vi "PhotonPipelineResult_Unpack.vi"(11 "RawData":u8[](array[numeric])) -> (3 "PhotonPipelineResult_REF":T1)   [LabVIEW 2019, in "PhotonVisionLib.lvlib"]
doc: "Internal function to parse the data returned by PhotonCamera_GetLatestResult.\n\nInputs:\n - RawData -- Byte array containing the data to parse.\n\nOutputs:\n - PipelineResult -- Parsed PipelineResult cluster."
uses:
  PhotonVisionLib.lvlib
  TargetCorner_New.vi
  Packet_decode_Int32.vi
  Packet_decode_Transform3d.vi
  PhotonPNPResult_unpackt.vi
  PhotonMultiTargetPNPResult_New.vi
  PhotonMultiTargetPNPResult_MAX_IDS.vi
  Packet_decode_Int16.vi
  <vilib>/Rock Robotics/WPI/ThirdParty/JAS_Junk/TrajLib/VI/Transform3d_Create_Trans3dRot3d.vi
  <vilib>/Rock Robotics/WPI/ThirdParty/JAS_Junk/TrajLib/VI/Translation3d_Create.vi
  <vilib>/Rock Robotics/WPI/ThirdParty/JAS_Junk/TrajLib/VI/Rotation3d_Create_Quaternion.vi
  <vilib>/Rock Robotics/WPI/ThirdParty/JAS_Junk/TrajLib/VI/Quaternion_New.vi
  Packet_decode_Boolean.vi
  PhotonPNPResult_New_Empty.vi
  PhotonPNPResult_New.vi
  <vilib>/Rock Robotics/WPI/ThirdParty/JAS_Junk/TrajLib/VI/Quaternion_Normalize.vi
  <vilib>/Rock Robotics/WPI/ThirdParty/JAS_Junk/TrajLib/VI/Quaternion_New_Default.vi
  TypeDef/TargetCornerType.ctl
  TypeDef/PhotonTrackedTargetType.ctl
  <vilib>/Rock Robotics/WPI/ThirdParty/JAS_Junk/TrajLib/TypeDef/QUATERNION.ctl
  <vilib>/Rock Robotics/WPI/ThirdParty/JAS_Junk/TrajLib/Trajectory_Library.lvlib
  <vilib>/Rock Robotics/WPI/ThirdParty/JAS_Junk/TrajLib/TypeDef/ROTATION3D.ctl
  <vilib>/Rock Robotics/WPI/ThirdParty/JAS_Junk/TrajLib/TypeDef/TRANSLATION3D.ctl
  <vilib>/Rock Robotics/WPI/ThirdParty/JAS_Junk/TrajLib/TypeDef/TRANSFORM3D.ctl
  TypeDef/PhotonPNPResultType.ctl
  TypeDef/PhotonMultiTargetPNPResultType.ctl
  TypeDef/PhotonPipelineResultType.ctl
  Ref/PhotonPipelineResult_REF.ctl
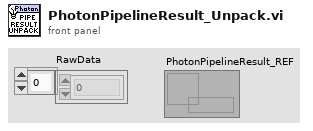
[diagram p1: front panel]
types:
  T1 = typedef "PhotonVisionLib.lvlib/PhotonPipelineResult_REF.ctl" = refnum<data-value>
  T2 = typedef "PhotonVisionLib.lvlib/PhotonMultiTargetPNPResultType.ctl" = cluster{"PhotonPNPResult":T3, "FiducialIDsUsed":i16[]}
  T3 = typedef "PhotonVisionLib.lvlib/PhotonPNPResultType.ctl" = cluster{"IsPresent":bool, "bestReprojErr":dbl, "altReprojErr":dbl, "ambiguity":dbl, "Best":T4, "Alt":T4}
  T4 = typedef "Trajectory_Library.lvlib/TRANSFORM3D.ctl" = cluster{"TRANSLATION3D":T5, "ROTATION3D":T6, "XF":bool}
  T5 = typedef "Trajectory_Library.lvlib/TRANSLATION3D.ctl" = cluster{"X":dbl, "Y":dbl, "Z":dbl}
  T6 = typedef "Trajectory_Library.lvlib/ROTATION3D.ctl" = cluster{"Q_quaternion":T7}
  T7 = typedef "Trajectory_Library.lvlib/QUATERNION.ctl" = cluster{"R":dbl, "V":dbl[]}
  T8 = typedef "PhotonVisionLib.lvlib/PhotonTrackedTargetType.ctl" = cluster{"Yaw":dbl, "Pitch":dbl, "Area":dbl, "Skew":dbl, "MinAreaRectCorners":T9[], "BestCameraToTarget":T4, "FiiducialId":i32, "AltCameraToTarget":T4, "PoseAmbiguity":dbl, "DetectedCorners":T9[]}
  T9 = typedef "PhotonVisionLib.lvlib/TargetCornerType.ctl" = cluster{"X":dbl, "Y":dbl}
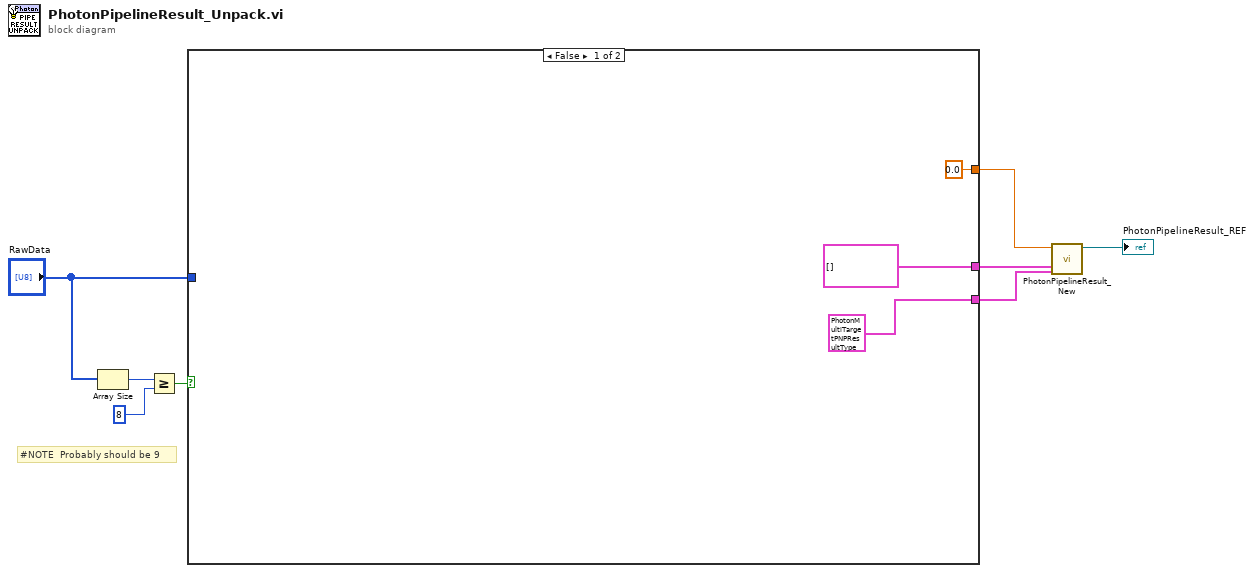
[diagram p0: block diagram]
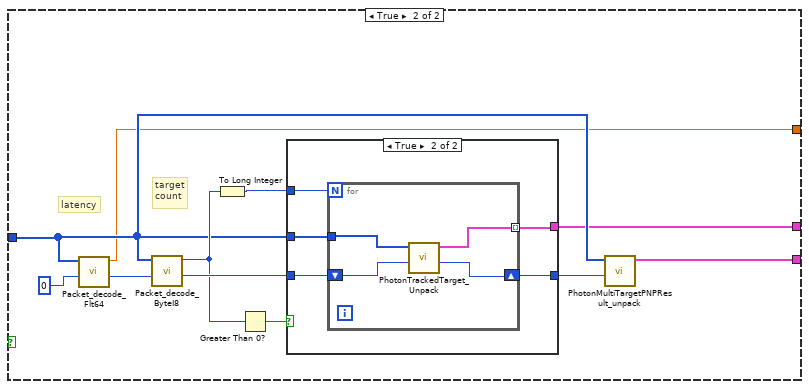
[diagram p2: hidden frame]
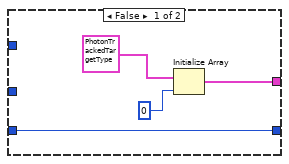
[diagram p3: hidden frame]
diagram:
  # "#NOTE  Probably should be 9"
  n1 = Array Size(array="RawData") -> (size(s)=w7:i32)
  n2 = Greater Or Equal?(x=w7, y=8) -> (x >= y?=w8:bool)
  n3 = case shown="False" w8 {
    tunnel: "RawData" -> [_ w15]
    tunnel: [T2 {"PhotonPNPResult"={"IsPresent"=FALSE, "bestReprojErr"=0.0, "altReprojErr"=0.0, "ambiguity"=0.0, "Best"={"TRANSLATION3D"={"X"=0.0, "Y"=0.0, "Z"=0.0}, "ROTATION3D"={"Q_quaternion"={"R"=1.0, "V"=[0.0, 0.0, 0.0]}}, "XF"=FALSE}, "Alt"={"TRANSLATION3D"={"X"=0.0, "Y"=0.0, "Z"=0.0}, "ROTATION3D"={"Q_quaternion"={"R"=1.0, "V"=[0.0, 0.0, 0.0]}}, "XF"=FALSE}}, "FiducialIDsUsed"=[]} ("MultiTargetPNP_Result") w14] -> w4
    tunnel: [T8[] [] w13] -> w3
    tunnel: [0.0 ("Flt64_Value") w12] -> w2
    frame False {
    }
    frame True {
      # "target\ncount"
      # "latency"
      n4 = call "Packet_decode_Flt64.vi"("StartByte"=0, "RawData"=w15) -> ("NextByte"=w17:i32, "Flt64_Value"=w12:dbl)  [unwired: 8 in]
      n5 = call "Packet_decode_ByteI8.vi"("StartByte"=w17, "RawData"=w15) -> ("NextByte"=w20:i32, "Int8_Value"=w19:i8)  [unwired: 8 in]
      n6 = To Long Integer(number=w19) -> (32bit integer=w18:i32)
      n7 = Greater Than 0?(x=w19) -> (x > 0?=w21:bool)
      n8 = case shown="True" w21 {
        tunnel: w20 -> [w23 w31]
        tunnel: w15 -> [_ w30]
        tunnel: w18 -> [_ w29]
        tunnel: [w24 w28] -> w13
        tunnel: [w23 w27] -> w16
        frame False {
          n9 = Initialize Array(T8 {"Yaw"=0.0, "Pitch"=0.0, "Area"=0.0, "Skew"=0.0, "MinAreaRectCorners"=[], "BestCameraToTarget"={"TRANSLATION3D"={"X"=0.0, "Y"=0.0, "Z"=0.0}, "ROTATION3D"={"Q_quaternion"={"R"=1.0, "V"=[0.0, 0.0, 0.0]}}, "XF"=FALSE}, "FiiducialId"=0, "AltCameraToTarget"={"TRANSLATION3D"={"X"=0.0, "Y"=0.0, "Z"=0.0}, "ROTATION3D"={"Q_quaternion"={"R"=1.0, "V"=[0.0, 0.0, 0.0]}}, "XF"=FALSE}, "PoseAmbiguity"=0.0, "DetectedCorners"=[]} ("PhotonTrackedTarget"), 0 ("dimension size")) -> (w24:T8[])
        }
        frame True {
          n10 = for {
            N: w29 -> [_]
            shift-right: [w32] -> w27
            shift-left: w31 -> [w34]
            tunnel: w30 -> [w35]
            tunnel: [w33] -> w28 mode=indexing
            n11 = call "PhotonTrackedTarget_Unpack.vi"("StartByte"=w34, "RawData"=w35) -> ("NextByte"=w32:i32, "TrackedTarget"=w33:T8)  [unwired: 8 in]
          }
        }
      }
      n12 = call "PhotonMultiTargetPNPResult_unpack.vi"("StartByte"=w16, "RawData"=w15) -> ("MultiTargetPNP_Result"=w14:T2)  [unwired: 8 in, 1 out]
    }
  }
  n13 = call "PhotonPipelineResult_New.vi"("PhotonMultiTargetPNPResult"=w4, "TrackedTargets"=w3, "Latency_Millis"=w2) -> ("PhotonPipelineResult_REF"=→"PhotonPipelineResult_REF":T1)  [unwired: 8 in]
